vi "Debug.vi"() -> ()   [LabVIEW 2020]
uses:
  <instrlib>/Marlin Instrument Driver/Public/controls/temperatures.ctl
  <instrlib>/Marlin Instrument Driver/Marlin Instrument Driver.lvlib
panel:
  out "Temperatures":T1
  in  "VISA resource name":refnum<visa-resource-name>="COM4"
  in  "Action Button":bool
  in  "stop":bool
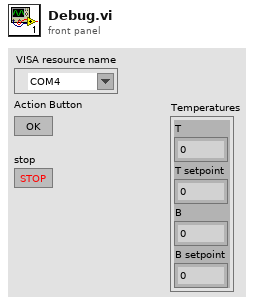
[diagram p1: front panel]
types:
  T1 = typedef "Marlin Instrument Driver.lvlib/temperatures.ctl" = cluster{"T":dbl, "T setpoint":dbl, "B":dbl, "B setpoint":dbl}
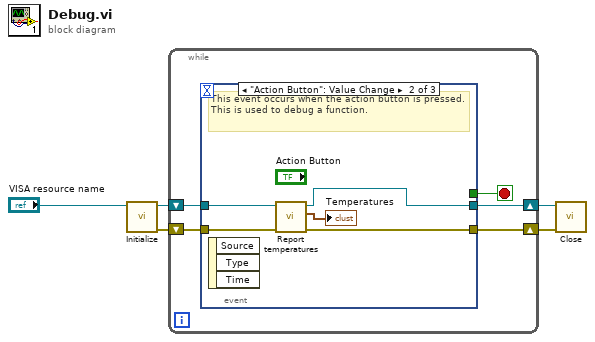
[diagram p0: block diagram]
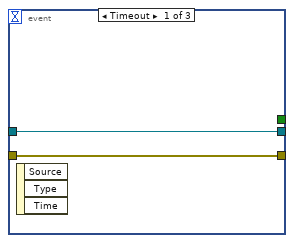
[diagram p2: hidden frame]
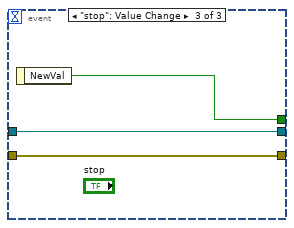
[diagram p3: hidden frame]
diagram:
  n1 = call <instrlib>:"Initialize.vi"("VISA resource name"="VISA resource name") -> ("error out"=w5:errorcluster, "VISA resource name out"=w4:refnum<visa-resource-name>)  [unwired: 9 in]
  n2 = while {
    shift-right: [w8] -> w2
    shift-left: w5 -> [w10]
    shift-right: [w7] -> w3
    shift-left: w4 -> [w9]
    stop <- w6 stop-if-true
    n3 = event shown="[1] \"Action Button\": Value Change" {
      selector: _ -> [_ _ _]
      dyn-events: _ -> [_ _ _]
      timeout: _ -> [_ _ _]
      tunnel: w10 -> [w11 w17 w18]
      tunnel: w9 -> [w12 w16 w19]
      tunnel: [w11 w15 w18] -> w8
      tunnel: [w12 w14 w19] -> w7
      tunnel: [_ _ w20] -> w6
      event Timeout {
        n4 = event-data() -> ()  [unwired: 1 in, 3 out]
      }
      event "Action Button": Value Change {
        # "This event occurs when the action button is pressed. This is used to debug a function."
        n5 = event-data() -> ()  [unwired: 1 in, 3 out]
        n6 = call <instrlib>:"Report temperatures.vi"("error in (no error)"=w17, "VISA resource name"=w16) -> ("error out"=w15:errorcluster, "Temperatures"=→"Temperatures":T1, "VISA resource name out"=w14:refnum<visa-resource-name>)  [unwired: 7 in]
      }
      event "stop": Value Change {
        n7 = event-data() -> ("NewVal"=w20:bool)  [unwired: 1 in]
      }
    }
  }
  n8 = call <instrlib>:"Close.vi"("error in (no error)"=w2, "VISA resource name"=w3) -> ()  [unwired: 9 in, 1 out]
